vi "jfcRigControlOnly_v8.vi"() -> ()   [LabVIEW 2018]
doc: "The Low-Level Grab VI configures the number of buffers to use for the acquisition and configures an event callback to handle every other acquired image. A grab is appropriate for high-speed applications in which you need to process only one image at a time."
uses:
  jfcStateEnumWithBeep.ctl
  jfcOptoStateEnum.ctl
  65be267c-4a08-44b7-a786-4a83c3a2bfd1.vi
  <vilib>/DAQmx/write.llb/DAQmx Write (Digital Bool 1Line 1Point).vi
  <vilib>/DAQmx/write.llb/DAQmx Write (Analog 1D DBL 1Chan NSamp).vi
  <vilib>/DAQmx/read.llb/DAQmx Read (Analog 1D Wfm NChan NSamp).vi
  <vilib>/DAQmx/write.llb/DAQmx Write (Analog Wfm 1Chan NSamp).vi
  <vilib>/DAQmx/configure/timing.llb/DAQmx Timing (Sample Clock).vi
  <vilib>/Instr/_visa.llb/VISA Configure Serial Port (Instr).vi
  <vilib>/DAQmx/create/channels.llb/DAQmx Create Channel (DO-Digital Output).vi
  <vilib>/DAQmx/miscellaneous.llb/DAQmx Fill In Error Info.vi
  <vilib>/DAQmx/create/channels.llb/DAQmx Create Channel (CO-Pulse Generation-Frequency).vi
  <vilib>/DAQmx/configure/timing.llb/DAQmx Timing (Implicit).vi
  <vilib>/Waveform/WDTOps.llb/WDT Append Waveforms DBL.vi
  <resource>/objmgr/daqmx.rc
  <vilib>/measure/NI_MABase.lvlib
panel:
  out "State":T1
  in  "amplitude":dbl=2.0 step=0.5 format="%#_13g"
  in  "rampUpOpto":bool
  in  "optoMaxTime":dbl=60.0 format="%.1g"
  in  "opto every trial?":bool
  in  "InhOptoOffset":dbl=2.3 step=0.5 format="%#_13g"
  out "platformExtended":bool
  out "opto time":dbl
  out "trial / jump #":i32
  out "opto trial list":bool[](array[boolean])
  in  "seconds to wait at end":i32=30
  in  "manual opto ON\n(overides enable)":bool
  in  "Opto-inhibition \nwaveform?":bool=TRUE
  out "BeepOn":bool
  out "beepTimeCurrent":u32 caption="Elapsed Time (s)"
  out "beepTimeElapsed":bool caption="Time has Elapsed"
  out "Waveform Graph":waveform(dbl)(graph) caption="Optostim waveform"
  out "optostim on":bool
  out "cold air status":bool
  out "session time elapsed":bool
  in  "seconds to wait at beg":i32=30
  in  "constant seconds to wait":u32=10
  out "seconds elapsed":i32
  out "Waveform Chart":waveform(dbl)[](graph)=[{"t0"=timestamp(3694175544.180511 s since 1904-01-01), "dt"=9.999999999999999e-05, "Y"=[2.549736107551297, 2.547978168445268, 2.549816013874609, 2.5507748897564566, 2.5496562012280126, 2.548697325350701, 2.5489370443196644, 2.5513342340226637, 2.550934702403809, 2.54845760638198, 2.548697325350701, 2.5504552644620753, 2.5508547960801193, 2.549736107551297, 2.54845760638198, 2.549176763288871, 2.551893578290195, 2.550615077109212, 2.547978168445268, 2.5492566696119936], "attributes"=variant("NI_ChannelName"=variant(string "jumpVoltageInput6281"), "NI_UnitDescription"=variant(string "Volts"))}]
  out "# frames triggered":i32
  in  "seconds to record":i32=1200
  in  "Frames Per Second":dbl=400.0 format="%.1f"
  out "numSamplesAvg":i32=20
  in  "jumpThresh":dbl=2.8000000000000003 step=0.01 format="%_3g"
  in  "manual solenoid override":bool
  out "beenStopped":bool=TRUE
  in  "ExtensionLength (mm)":dbl=100.0 caption="Extension Length (mm)"
  out "jump voltage":dbl=2.549672182495309 format="%#_3g"
  in  "optostim enable":bool=TRUE
  out "error out":errorcluster={"status"=FALSE, "code"=1073676294, "source"="VISA Read in usbSimpleRelayCommand.vi->jfcRigControlOnly_v3_constantTimingWithBeep.vi"}
  in  "stop":bool
  # "optostim Enable"
  # "[change # frames \nin video program too]"
  # "----------------------------------------------------------------------------------------------------------------------------"
  # "5"
  # "10"
  # "15"
  # "20"
  # "25"
  # "30"
  # "35"
  # "40"
  # "45"
  # "50"
  # "55"
  # "60"
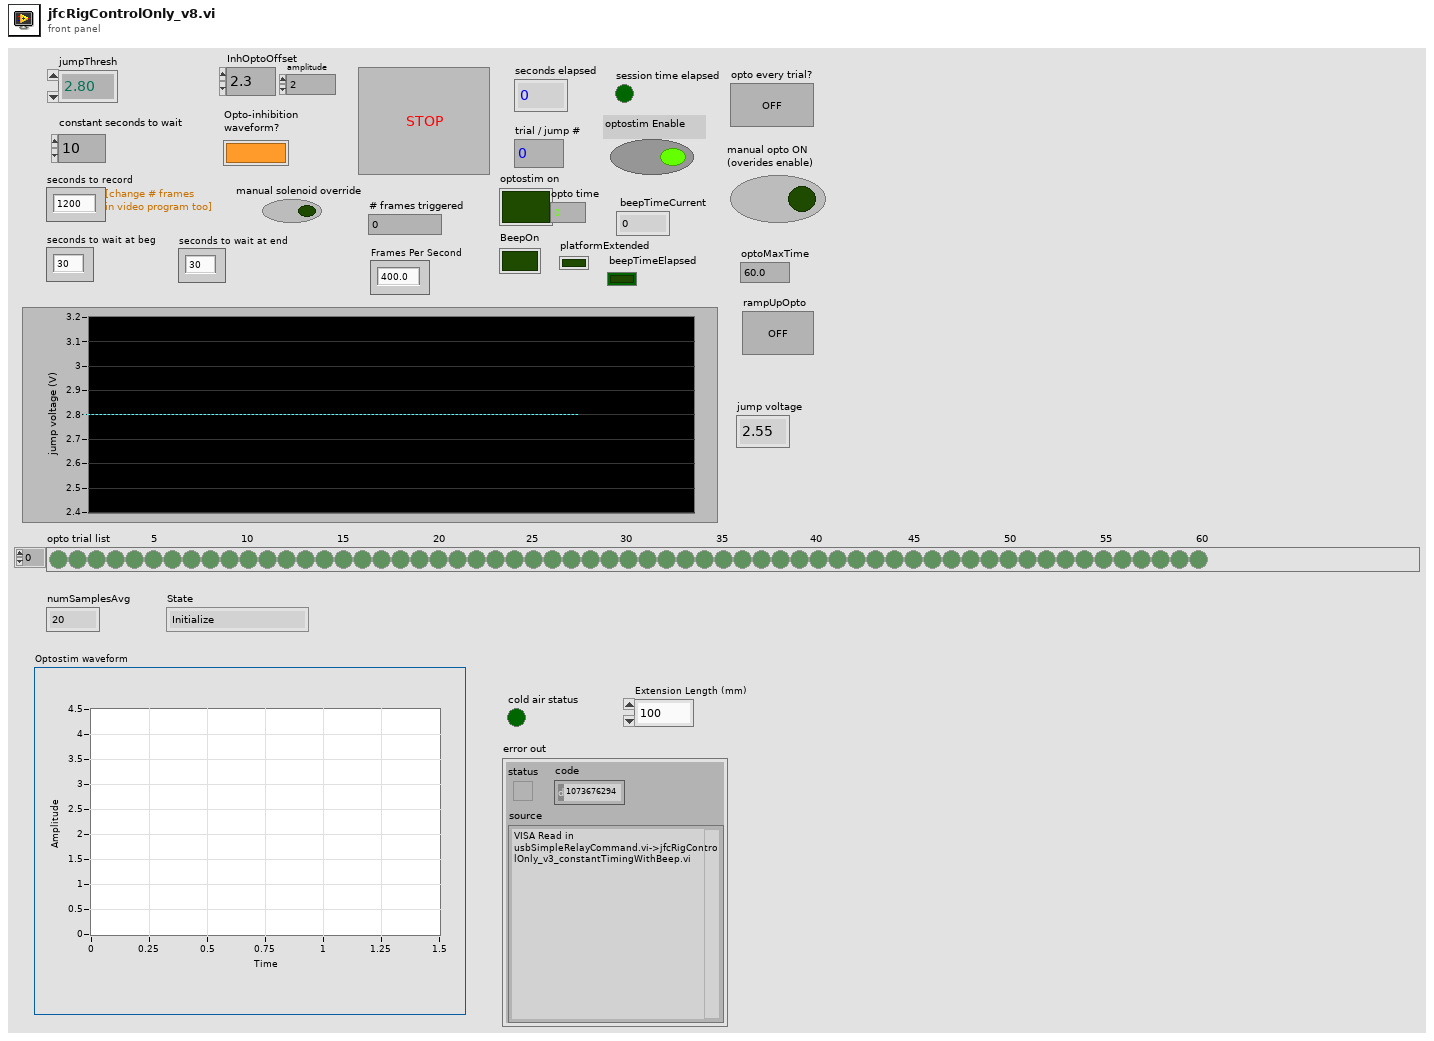
[diagram p1: front panel]
types:
  T1 = typedef "jfcStateEnumWithBeep.ctl" = enum16{"Initialize", "Reinitialize after jump", "Beep", "Wait for Thresh or Stop", "Turn Off Air and Reset Lever", "Wait after time elapsed", "Stop"}
  T2 = enum16{"Sine Wave", "Triangle Wave", "Square Wave", "Sawtooth Wave"}
  T3 = typedef "jfcOptoStateEnum.ctl" = enum16{"writeZeroVoltage", "WaitForStartOpto", "RampUpOpto", "OptoOn", "RampDownOpto"}
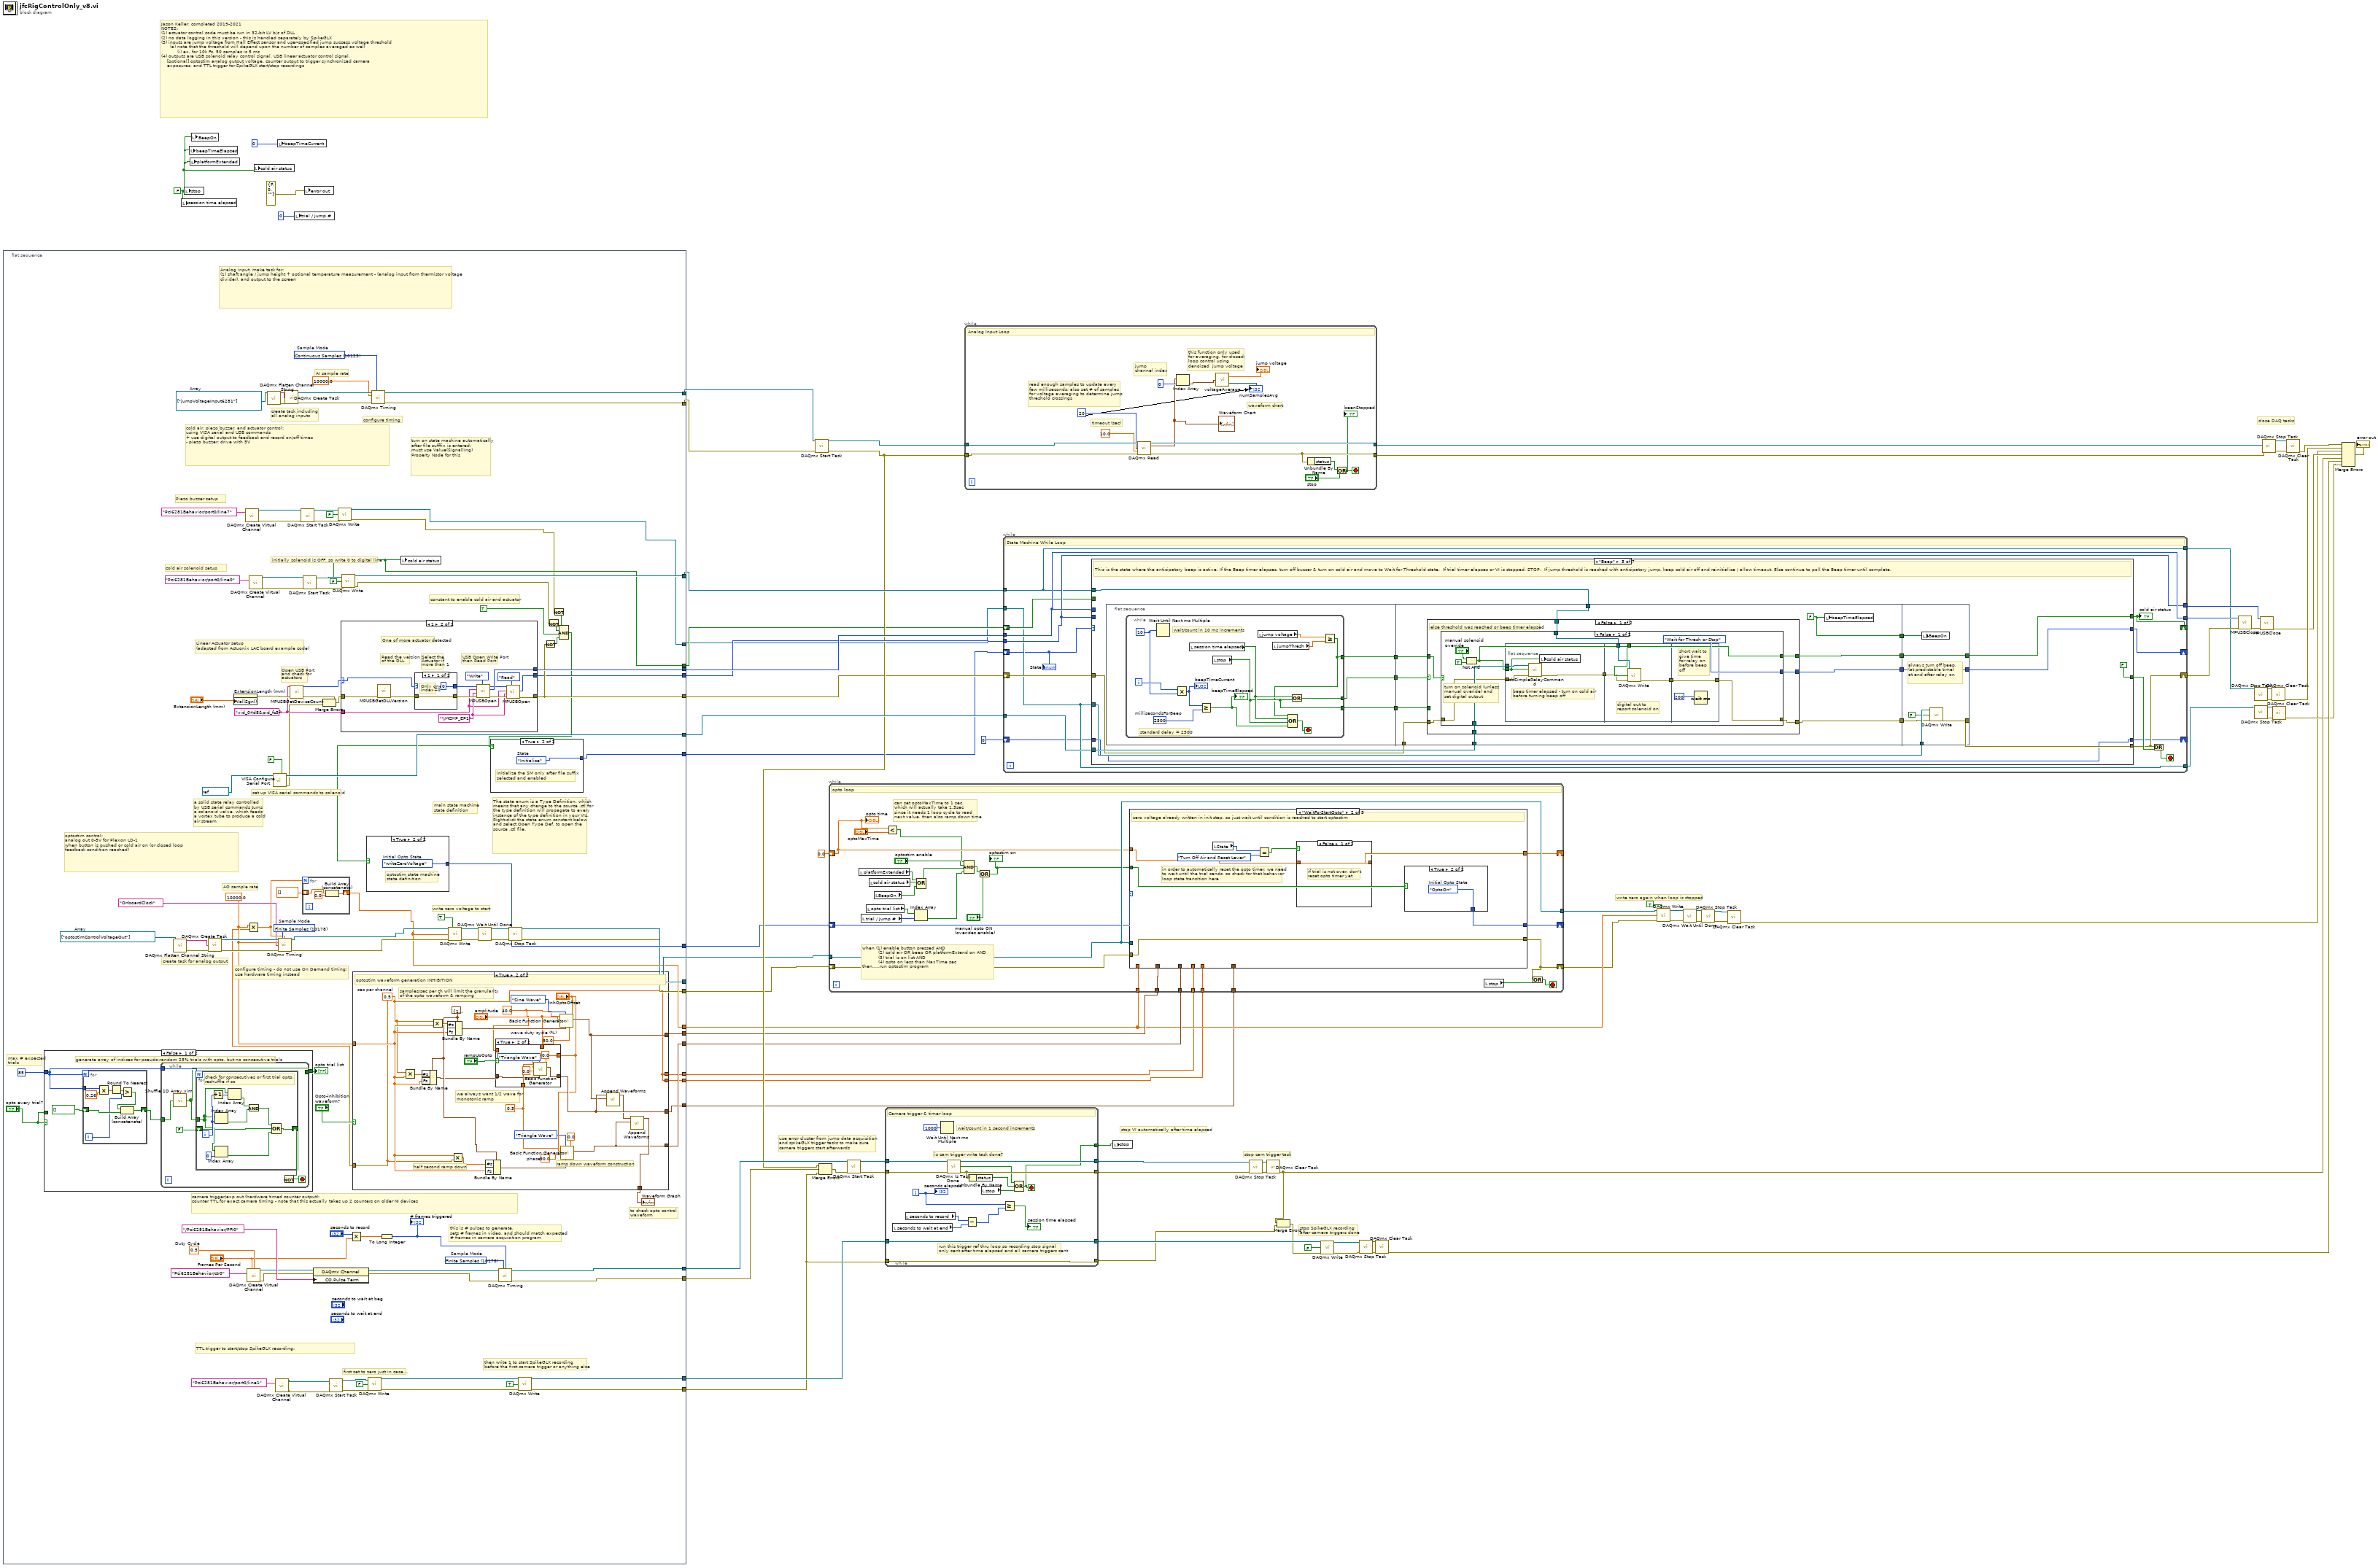
[diagram p0: block diagram]
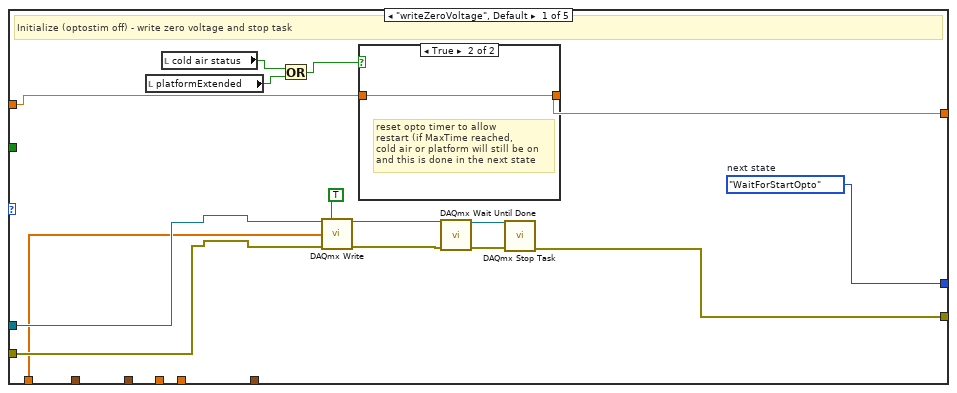
[diagram p2: hidden frame]
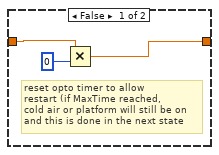
[diagram p3: hidden frame]
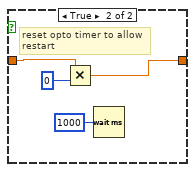
[diagram p4: hidden frame]
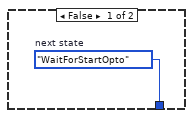
[diagram p5: hidden frame]
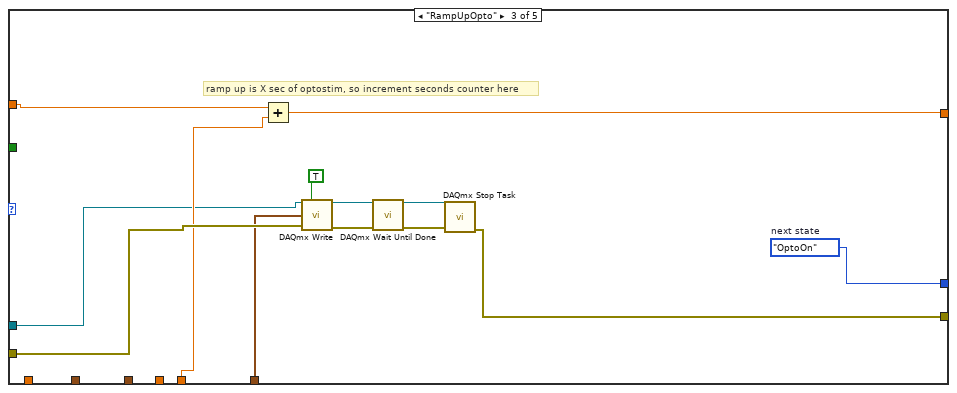
[diagram p6: hidden frame]
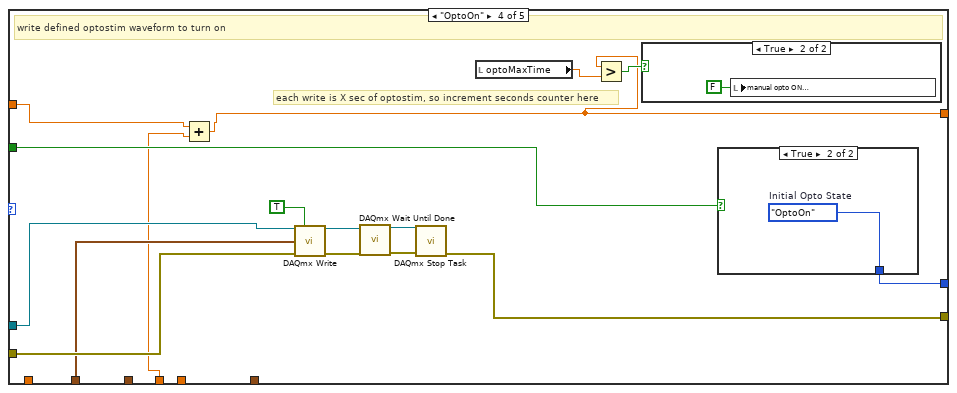
[diagram p7: hidden frame]
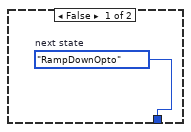
[diagram p9: hidden frame]
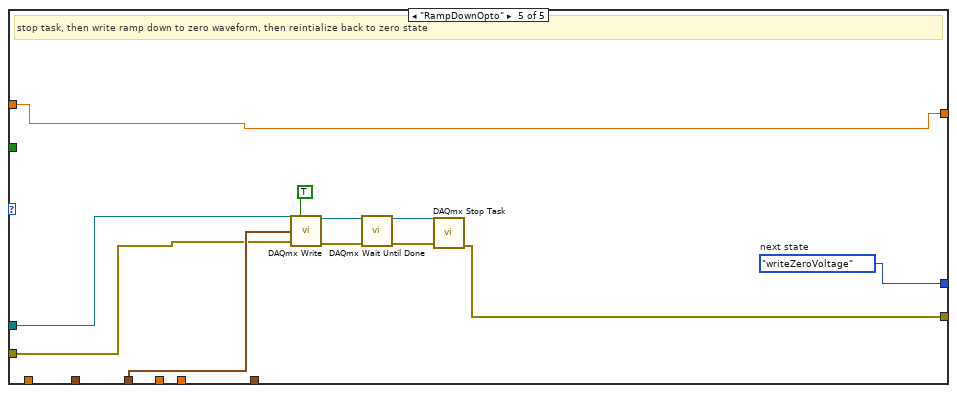
[diagram p10: hidden frame]
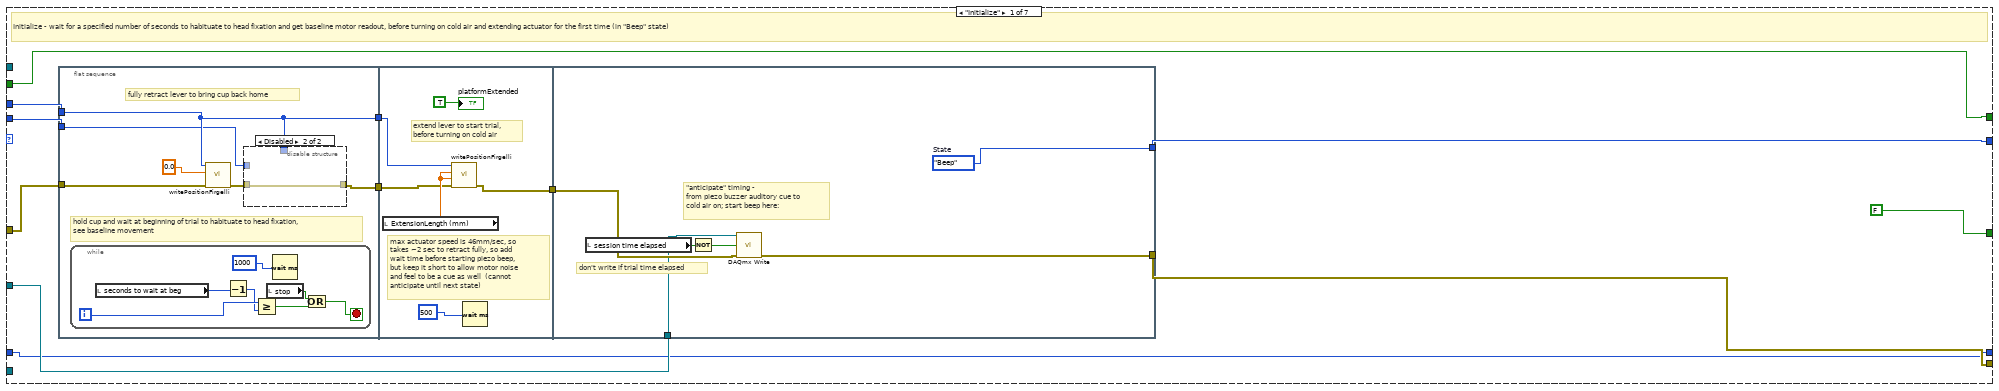
[diagram p11: hidden frame]
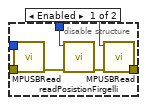
[diagram p12: hidden frame]
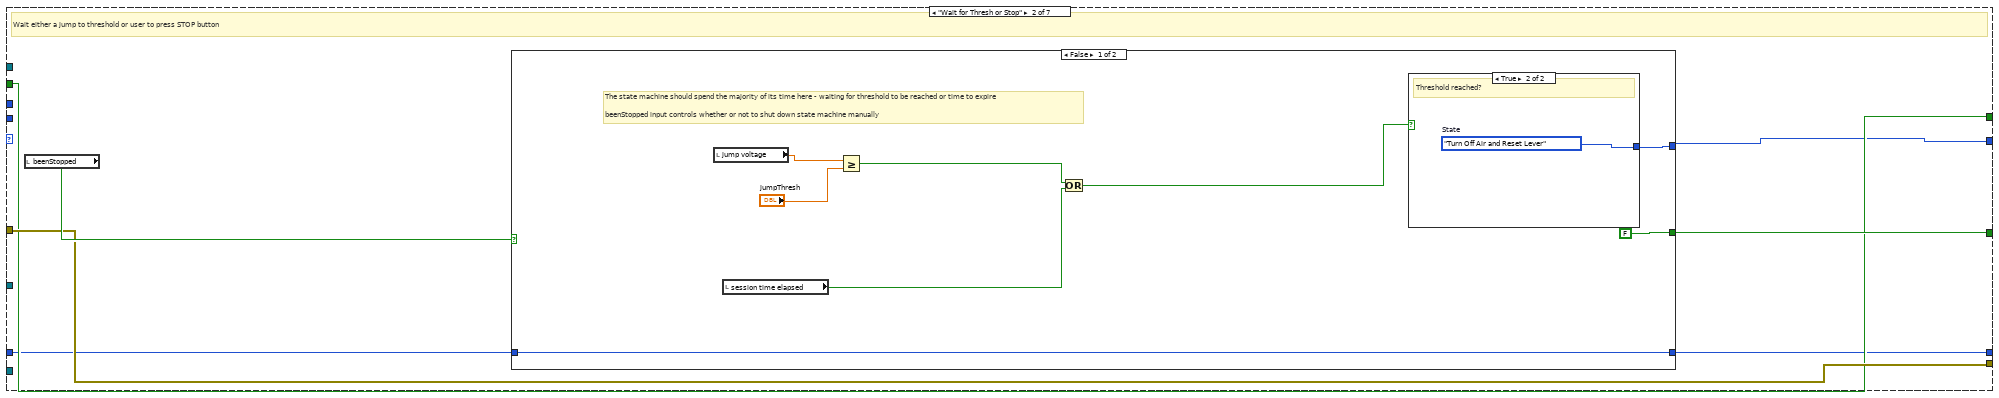
[diagram p13: hidden frame]
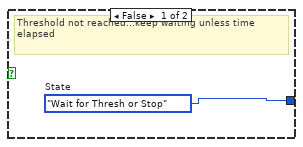
[diagram p14: hidden frame]
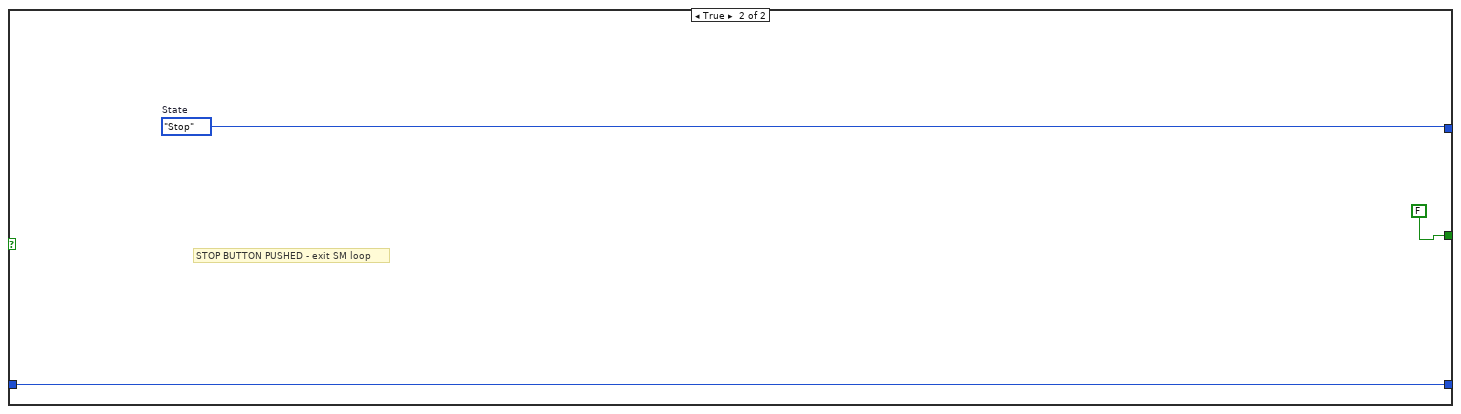
[diagram p15: hidden frame]
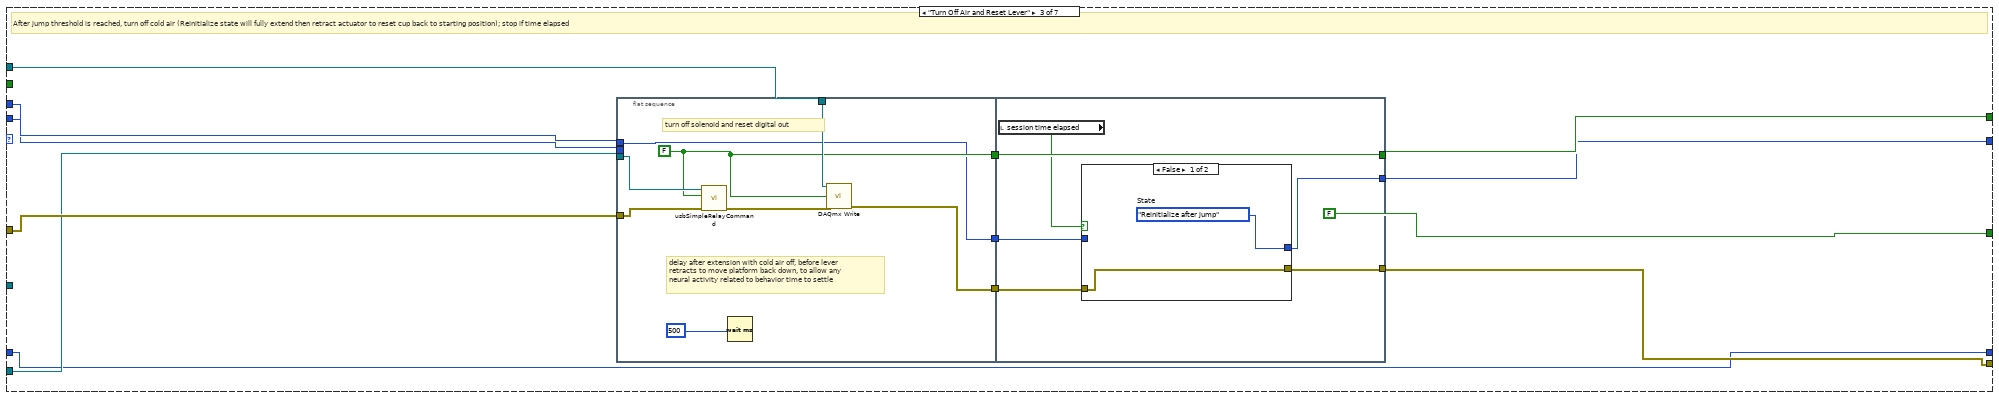
[diagram p16: hidden frame]
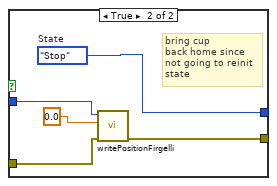
[diagram p17: hidden frame]
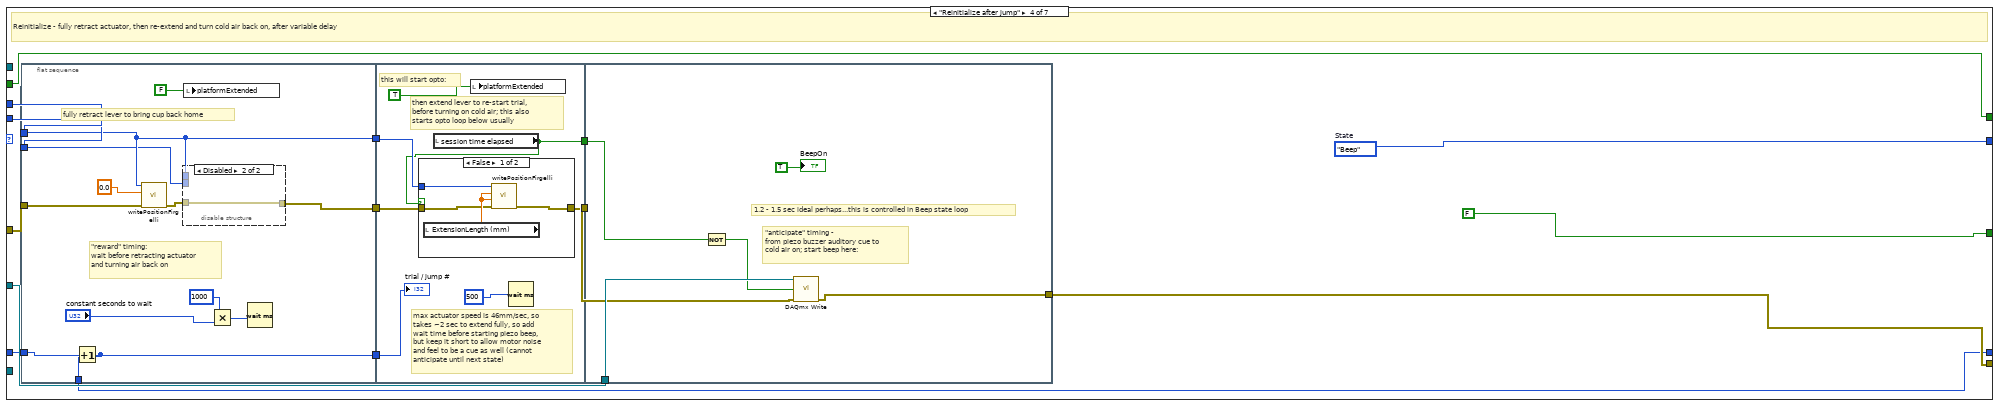
[diagram p18: hidden frame]
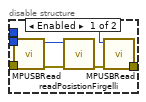
[diagram p19: hidden frame]
diagram:
  w4 = FALSE ("stop")
  # "stop cam trigger task"
  # "write zero again when loop is stopped"
  # "stop SpikeGLX recording\nafter camera triggers done"
  # "stop VI automatically after time elapsed"
  # "use error cluster from jump data acquisition\nand spikeGLX trigger tasks to make sure \ncamera triggers start afterwards"
  # "Jason Keller, completed 2019-2021\nNOTES: \n(1) actuator control code must be run in 32-bit LV b/c of DLL \n(2) no data logging in this version - this is handled separately by SpikeGLX\n(3) inputs are jump voltage from Hall Effect sensor and user-specified jump success voltage threshold\n      (a) note that the threshold will depend upon the number of samples averaged as well\n           (i) ex. for 10k Fs, 50 samples is 5 ms\n(4) outputs are USB solenoid relay control signal, USB linear actuator control signal, \n    [optional] optostim analog output voltage, counter output to trigger synchronized camera \n    exposures, and TTL trigger for SpikeGLX start/stop recordings"
  # "close DAQ tasks"
  n1 = flat-sequence {
    tunnel: [w150] -> w71
    tunnel: [w149] -> w70
    tunnel: [w162] -> w60
    tunnel: [w173] -> w19
    tunnel: [w168] -> w69
    tunnel: [w167] -> w48
    tunnel: [w165] -> w67
    tunnel: [w158] -> w59
    tunnel: [w136] -> w52
    tunnel: [w135] -> w50
    tunnel: [w134] -> w47
    tunnel: [w115] -> w44
    tunnel: [w92] -> w43
    tunnel: [w127] -> w46
    tunnel: [w126] -> w45
    tunnel: [w125] -> w40
    tunnel: [w117] -> w38
    tunnel: [w104] -> w36
    tunnel: [w103] -> w35
    tunnel: [w97] -> w24
    tunnel: [w89] -> w2
    tunnel: [w88] -> w3
    tunnel: [w87] -> w1
    frame #0 {
      w148 = 0.5  # Duty Cycle
      w128 = refnum<k21>[] ["optostimControlVoltageOut"]  # Array
      w86 = 10000.0 ("Sample Rate")
      w132 = 10178 items=["Finite Samples"=10178, "Continuous Samples"=10123, "Hardware Timed Single Point"=12522]  # Sample Mode
      w141 = 10178 items=["Finite Samples"=10178, "Continuous Samples"=10123, "Hardware Timed Single Point"=12522]  # Sample Mode
      w134 = FALSE ("data")
      w169 = "vid_04d8&pid_fc5f"
      w174 = refnum<k21>[] ["jumpVoltageInput6281"]  # Array
      w179 = 10123 items=["Finite Samples"=10178, "Continuous Samples"=10123, "Hardware Timed Single Point"=12522]  # Sample Mode
      # "max # expected\ntrials"
      # "to check opto control\nwaveform"
      # "cold air solenoid setup"
      # "Piezo buzzer setup"
      # "Piezo buzzer setup"
      # "then write 1 to start SpikeGLX recording\nbefore the first camera trigger or anything else"
      # "first set to zero just in case..."
      # "TTL trigger to start/stop SpikeGLX recording:"
      # "write zero voltage to start"
      # "AO sample rate"
      # "create task for analog output"
      # "configure timing - do not use On Demand timing; \nuse hardware timing instead"
      # "this is # pulses to generate,\nsets # frames in video, and should match expected \n# frames in camera acquisition program"
      # "camera trigger/exp out (hardware timed counter output): \ncounter TTL for exact camera timing - note that this actually takes up 2 counters on older NI devices"
      # "initially solenoid is OFF, so write 0 to digital line"
      # "set up VISA serial commands to solenoid"
      # "Linear Actuator setup\n(adapted from Actuonix LAC board example code)"
      # "Open USB Port\nand check for\nactuators"
      # "turn on state machine automatically\nafter file sufffix is entered;\nmust use Value(Signalling) \nProperty Node for this"
      # "The state enum is a Type Definition, which means that any change to the source .ctl for the type definition will propagate to every instance of the type definition in your VIs. Right-click the state enum constant below and select Open Type Def. to open the source .ctl file."
      # "main state machine\nstate definition"
      # "a solid state relay controlled\nby USB serial commands turns\na solenoid valve, which feeds\na vortex tube to produce a cold\nair stream"
      # "AI sample rate"
      # "create task including\nall analog inputs"
      # "configure timing"
      # "constant to enable cold air and actuator"
      # "optostim control: \nanalog out 0-5V for Plexon LD-1\nwhen button is pushed or cold air on (or closed loop \nfeedback condition reached)"
      # "Analog input, make task for:\n(1) shaft angle / jump height + optional temperature measurement - (analog input from thermistor voltage divider), and output to the screen"
      # "cold air, piezo buzzer, and actuator control: \nusing VISA serial and USB commands\n+ use digital output to feedback and record on/off times\n- piezo buzzer: drive with 5V"
      n2 = case shown="False" "opto every trial?" {
        tunnel: 85 -> [w182 w212]
        tunnel: [w181 w208] -> w90
        tunnel: "opto every trial?" -> [_ w213]
        frame False {
          # "generate array of indices for pseudo-random 25% trials with opto, but no consecutive trials"
          n3 = for {
            N: w182 -> [_]
            shift-right: [w188] -> w183
            shift-left: bool[] [] -> [w189]
            tunnel: w182 -> [w191]
            i -> [w184]
            n4 = Multiply(x=w191, y=0.26) -> (x*y=w186:dbl)
            n5 = Round To Nearest(number=w186) -> (nearest integer value=w185:dbl)
            n6 = Greater?(x=w185, y=w184) -> (0:w190:bool)
            n7 = Build Array (concatenate)(w190, w189) -> (w188:bool[])
          }
          n8 = while {
            tunnel: w183 -> [w197]
            tunnel: w182 -> [w196]
            tunnel: [w192] -> w181
            stop <- w194 stop-if-true
            n9 = call "Shuffle 1D Array.vim"("array"=w197) -> ("shuffled array"=w192:bool[])  [unwired: 4 in]
            n10 = for {
              N: w196 -> [_]
              tunnel: w192 -> [w202]
              shift-right: [w200] -> w193
              shift-left: FALSE -> [w201]
              i -> [w206]
              # "check for consecutives or first trial opto, \nreshuffle if so"
              n11 = Increment(x=w206) -> (x+1=w207:i32)
              n12 = Index Array(array=w202, index=w206) -> (element=w204:bool)
              n13 = Index Array(array=w202, index=0) -> (element=w198:bool)
              n14 = Index Array(array=w202, index=w207) -> (element=w205:bool)
              n15 = And(x=w205, y=w204) -> (x .and. y?=w199:bool)
              n16 = Compound Arithmetic op=OR(w199, w201, w198) -> (w200:bool)
            }
            n17 = Not(x=w193) -> (.not. x?=w194:bool)
          }
        }
        frame True {
          # "all trials except for #0"
          n18 = Decrement(x=w212) -> (x-1=w211:i32)
          n19 = Initialize Array(w213, w211) -> (w209:bool[])
          n20 = Build Array (concatenate)(FALSE, w209) -> (w208:bool[])
        }
      }
      "opto trial list" <- w90
      n21 = call <vilib>:"DAQmx Flatten Channel String.vi"("names in"=w128) -> ("names out"=w129:string, "error out"=w130:errorcluster)  [unwired: 13 in]
      n22 = call <vilib>:"DAQmx Create Task.vi"("global virtual channels"=w129, "error in"=w130) -> ("task out"=w131:refnum<k21>, "error out"=w93:errorcluster)  [unwired: 12 in]
      n23 = property on="ExtensionLength (mm)" class="DigNum (strict)"("Val(Sgnl)"="ExtensionLength (mm)") -> (error out=w172:errorcluster)  [unwired: 2 in, 1 out]
      n24 = call-poly <vilib>:"DAQmx Create Virtual Channel.vi"("lines"=tag "Pci6281Behavior/port0/line7") -> ("task out"=w82:refnum<k21>, "error out"=w81:errorcluster)  [unwired: 13 in]
      n25 = call-poly <vilib>:"DAQmx Create Virtual Channel.vi"("frequency"="Frames Per Second", "duty cycle"=w148, "counter"=tag "Pci6281Behavior/ctr0" ("Counter")) -> ("task out"=w143:refnum<k21>, "error out"=w144:errorcluster)  [unwired: 11 in]
      n26 = call-poly <vilib>:"DAQmx Create Virtual Channel.vi"("lines"=tag "Pci6281Behavior/port0/line0") -> ("task out"=w80:refnum<k21>, "error out"=w79:errorcluster)  [unwired: 13 in]
      n27 = call <vilib>:"DAQmx Flatten Channel String.vi"("names in"=w174) -> ("names out"=w175:string, "error out"=w176:errorcluster)  [unwired: 13 in]
      n28 = call-poly "VISA Configure Serial Port"("VISA resource name"=refnum<visa-resource-name> "COM4" ("relay COM port"), "Enable Termination\nChar (T)"=FALSE ("Enable Termination\nChar (T)")) -> ("VISA resource name out"=w162:refnum<visa-resource-name>, "error out"=w161:errorcluster)  [unwired: 12 in]
      n29 = call-poly <vilib>:"DAQmx Create Virtual Channel.vi"("lines"=tag "Pci6281Behavior/port0/line1") -> ("task out"=w111:refnum<k21>, "error out"=w110:errorcluster)  [unwired: 13 in]
      n30 = call <vilib>:"DAQmx Create Task.vi"("global virtual channels"=w175, "error in"=w176) -> ("task out"=w178:refnum<k21>, "error out"=w177:errorcluster)  [unwired: 12 in]
      n31 = call "MPUSBGetDeviceCount.vi"("error in (no error)"=w172, "pVID_PID"=w169) -> ("error out"=w160:errorcluster, "return_value"=w171:u32)  [unwired: 8 out]
      n32 = call <vilib>:"DAQmx Start Task.vi"("task/channels in"=w82, "error in"=w81) -> ("task out"=w98:refnum<k21>, "error out"=w101:errorcluster)  [unwired: 12 in]
      n33 = call <vilib>:"DAQmx Start Task.vi"("task/channels in"=w80, "error in"=w79) -> ("task out"=w154:refnum<k21>, "error out"=w153:errorcluster)  [unwired: 12 in]
      n34 = property class="DAQmx Channel"(reference=w143, error in=w144, "CO.Pulse.Term"=tag "/Pci6281Behavior/PFI0" ("Output Terminal")) -> (reference out=w147:refnum<k21>, error out=w146:errorcluster)
      n35 = Merge Errors(w160, w161) -> (w159:errorcluster)
      n36 = call <vilib>:"DAQmx Start Task.vi"("task/channels in"=w111, "error in"=w110) -> ("task out"=w113:refnum<k21>, "error out"=w112:errorcluster)  [unwired: 12 in]
      n37 = call-poly <vilib>:"DAQmx Write.vi"("task/channels in"=w98, "data"=FALSE, "error in"=w101) -> ("task out"=w97:refnum<k21>, "error out"=w96:errorcluster)  [unwired: 10 in, 1 out]
      n38 = case shown="1" w171 {
        selector: w171 -> [_ w282]
        tunnel: w159 -> [w272 w284]
        tunnel: w169 -> [_ w278]
        tunnel: [u32 0 ("HANDLE") w283] -> w168
        tunnel: [w272 w277] -> w167
        tunnel: [u32 0 ("HANDLE") w276] -> w165
        frame 0, Default {
          # "No actuator detected"
        }
        frame 1 {
          w279 = "\\MCHP_EP1" ("pEP")
          # "One of more actuator detected"
          # "Select the\nActuator if\nmore than 1"
          # "Read the version\nof the DLL"
          # "USB Open Write Port\nthen Read Port"
          n39 = call "MPUSBGetDLLVersion.vi"("error in (no error)"=w284) -> ("error out"=w287:errorcluster)  [unwired: 10 out]
          n40 = case shown="1" w282 {
            selector: w282 -> [_ w291]
            tunnel: w287 -> [w290 w294]
            tunnel: [w290 w293] -> w286
            tunnel: [u32 0 ("Selected") w292] -> w285
            frame 1 {
              # "Only one\nIndex=0"
            }
            frame Default {
              n41 = call "actuatorSelect.vi"("error in (no error)"=w294, "Devices"=w291) -> ("error out"=w293:errorcluster, "Selected"=w292:u32)  [unwired: 8 out]
            }
          }
          n42 = call "MPUSBOpen.vi"("dwDir"=enum16{"Write", "Read"}."Write", "error in (no error)"=w286, "pEP"=w279, "pVID_PID"=w278, "instance"=w285) -> ("error out"=w280:errorcluster, "HANDLE"=w283:u32, "instanceOut"=w275:u32)  [unwired: 4 in]
          n43 = call "MPUSBOpen.vi"("dwDir"=enum16{"Write", "Read"}."Read", "error in (no error)"=w280, "pEP"=w279, "pVID_PID"=w278, "instance"=w275) -> ("error out"=w277:errorcluster, "HANDLE"=w276:u32)  [unwired: 3 in, 2 out]
        }
      }
      n44 = call-poly <vilib>:"DAQmx Write.vi"("task/channels in"=w154, "data"=w134, "error in"=w153) -> ("task out"=w158:refnum<k21>, "error out"=w157:errorcluster)  [unwired: 10 in, 1 out]
      n45 = Multiply(x="seconds to record", y="Frames Per Second") -> (x*y=w138:dbl)
      n46 = case shown="True" "Opto-inhibition \nwaveform?" {
        tunnel: w86 -> [w222 w240]
        tunnel: [w227 w243] -> w126
        tunnel: [w224 w241] -> w125
        tunnel: [w225 w247] -> w94
        tunnel: [w217 w232] -> w89
        tunnel: [w217 w232] -> w88
        tunnel: [w228 w244] -> w87
        tunnel: [w217 w232] -> w84
        frame False {
          w217 = 0.5  # sec per channel
          w223 = 40.0 ("y")
          w218 = T2."Square Wave" ("signal type")
          w219 = 2.5  # amplitude
          w229 = 2.5  # offset
          w221 = 20.0  # square wave duty cycle (%)
          w220 = cluster{"Fs":dbl, "#s":dbl} {"Fs"=1000.0, "#s"=1000.0} ("sampling info")
          # "samples /sec per ch will limit the granularity\nof the opto waveform & ramping"
          # "excitation waveform\nex. 40Hz, 5ms pulse width"
          # "ex. 10ms/25ms = 0.4"
          # "optostim waveform generation EXCITATION"
          n47 = Multiply(x=w217, y=w222) -> (x*y=w231:dbl)
          n48 = Bundle By Name(cluster=w220, "#s"=w231, "Fs"=w222) -> (w230:cluster{"Fs":dbl, "#s":dbl})
          n49 = call <vilib>:"Basic Function Generator.vi"("offset"=w229, "square wave duty cycle (%)"=w221, "sampling info"=w230, "signal type"=w218, "amplitude"=w219, "frequency"=w223) -> ("signal out"=w227:waveform(dbl))  [unwired: 3 in, 2 out]
          n50 = call "buildRampDownWaveform.vi"("Fs"=w222, "square wave duty cycle (%)"=w221, "signal type"=w218, "input cluster"=w220, "amplitude"=w219, "freq"=w223, "sec rampdown"=w217) -> ("rampDown out"=w224:waveform(dbl))  [unwired: 4 in]
          n51 = call "buildRampUpWaveform.vi"("Fs"=w222, "square wave duty cycle (%)"=w221, "signal type"=w218, "input cluster"=w220, "amplitude"=w219, "freq"=w223, "sec rampup"=w217) -> ("rampUp out"=w228:waveform(dbl))  [unwired: 4 in]
          n52 = call-poly <vilib>:"Append Waveforms.vi"("waveform B"=w227, "waveform A"=w228) -> ("waveform out"=w226:waveform(dbl))  [unwired: 8 in, 1 out]
          n53 = call-poly <vilib>:"Append Waveforms.vi"("waveform B"=w224, "waveform A"=w226) -> ("waveform out"=w225:waveform(dbl))  [unwired: 8 in, 1 out]
        }
        frame True {
          w232 = 0.5  # sec per channel
          w234 = 0.5 ("frequency")
          w233 = 40.0 ("frequency")
          w254 = 90.0  # phase
          w255 = 50.0  # wave duty cycle (%)
          w246 = cluster{"Fs":dbl, "#s":dbl} {"Fs"=1000.0, "#s"=1000.0} ("sampling info")
          # "half second ramp down"
          # "samples/sec per ch will limit the granularity\nof the opto waveform & ramping"
          # "we always want 1/2 wave for\nmonotonic ramp"
          # "ramp down waveform construction"
          # "optostim waveform generation INHIBITION"
          n54 = Multiply(x=w232, y=w240) -> (x*y=w239:dbl)
          n55 = Bundle By Name(cluster=w246, "#s"=w239, "Fs"=w240) -> (w245:cluster{"Fs":dbl, "#s":dbl})
          n56 = Multiply(x=w232, y=w240) -> (x*y=w250:dbl)
          n57 = Bundle By Name(cluster=w246, "#s"=w250, "Fs"=w240) -> (w249:cluster{"Fs":dbl, "#s":dbl})
          n58 = Multiply(x=w240, y=w232) -> (x*y=w251:dbl)
          n59 = Bundle By Name(cluster=w246, "#s"=w251, "Fs"=w240) -> (w253:cluster{"Fs":dbl, "#s":dbl})
          n60 = case shown="True" "rampUpOpto" {
            tunnel: w245 -> [w262 w264]
            tunnel: [w260 w263] -> w244
            tunnel: "InhOptoOffset" -> [w258 w267]
            tunnel: "amplitude" -> [w257 _]
            tunnel: w233 -> [w256 _]
            tunnel: w234 -> [_ w269]
            frame False {
              w261 = 0.0  # phase
              n61 = call <vilib>:"Basic Function Generator.vi"("offset"=w258, "sampling info"=w262, "signal type"=T2."Sine Wave", "phase"=w261, "amplitude"=w257, "frequency"=w256) -> ("signal out"=w260:waveform(dbl))  [unwired: 3 in, 2 out]
            }
            frame True {
              n62 = call <vilib>:"Basic Function Generator.vi"("offset"=0.0, "sampling info"=w264, "signal type"=T2."Triangle Wave", "phase"=0.0, "amplitude"=w267, "frequency"=w269) -> ("signal out"=w263:waveform(dbl))  [unwired: 3 in, 2 out]
            }
          }
          n63 = call <vilib>:"Basic Function Generator.vi"("offset"="InhOptoOffset", "square wave duty cycle (%)"=w255, "sampling info"=w249, "signal type"=T2."Sine Wave", "amplitude"="amplitude", "frequency"=w233) -> ("signal out"=w243:waveform(dbl))  [unwired: 3 in, 2 out]
          n64 = call <vilib>:"Basic Function Generator.vi"("offset"=0.0, "sampling info"=w253, "signal type"=T2."Triangle Wave", "phase"=w254, "amplitude"="InhOptoOffset", "frequency"=w234) -> ("signal out"=w241:waveform(dbl))  [unwired: 3 in, 2 out]
          n65 = call-poly <vilib>:"Append Waveforms.vi"("waveform B"=w243, "waveform A"=w244) -> ("waveform out"=w242:waveform(dbl))  [unwired: 8 in, 1 out]
          n66 = call-poly <vilib>:"Append Waveforms.vi"("waveform B"=w241, "waveform A"=w242) -> ("waveform out"=w247:waveform(dbl))  [unwired: 8 in, 1 out]
        }
      }
      "Waveform Graph" <- w94
      n67 = Multiply(x=w86, y=w84) -> (x*y=w85:dbl)
      n68 = call-poly <vilib>:"DAQmx Timing.vi"("task/channels in"=w131, "sample mode"=w132, "samples per channel"=w85, "rate"=w86, "source"=tag "OnboardClock", "error in"=w93) -> ("task out"=w122:refnum<k21>, "error out"=w123:errorcluster)  [unwired: 8 in]
      n69 = for {
        N: w85 -> [_]
        shift-right: [w216] -> w117
        shift-left: dbl[] [] -> [w214]
        n70 = Build Array (concatenate)(w214, 0.0 ("element")) -> (w216:dbl[])
      }
      n71 = call-poly <vilib>:"DAQmx Write.vi"("task/channels in"=w113, "data"=FALSE, "error in"=w112) -> ("task out"=w106:refnum<k21>, "error out"=w105:errorcluster)  [unwired: 10 in, 1 out]
      n72 = call-poly <vilib>:"DAQmx Timing.vi"("task/channels in"=w178, "sample mode"=w179, "rate"=10000.0 ("Sample Rate"), "error in"=w177) -> ("task out"=w150:refnum<k21>, "error out"=w149:errorcluster)  [unwired: 10 in]
      n73 = To Long Integer(number=w138) -> (32bit integer=w137:i32)
      "# frames triggered" <- w137
      n74 = local write "cold air status"(w134) -> ()
      n75 = call-poly <vilib>:"DAQmx Write.vi"("task/channels in"=w122, "auto start"=TRUE, "data"=w117, "error in"=w123) -> ("task out"=w120:refnum<k21>, "error out"=w119:errorcluster)  [unwired: 9 in, 1 out]
      n76 = call <vilib>:"DAQmx Wait Until Done.vi"("task/channels in"=w120, "error in"=w119) -> ("task out"=w116:refnum<k21>, "error out"=w114:errorcluster)  [unwired: 12 in]
      n77 = call-poly <vilib>:"DAQmx Timing.vi"("task/channels in"=w147, "sample mode"=w141, "samples per channel"=w137, "error in"=w146) -> ("task out"=w135:refnum<k21>, "error out"=w136:errorcluster)  [unwired: 10 in]
      n78 = call <vilib>:"DAQmx Stop Task.vi"("task/channels in"=w116, "error in"=w114) -> ("task out"=w115:refnum<k21>, "error out"=w92:errorcluster)  [unwired: 12 in]
      n79 = call-poly <vilib>:"DAQmx Write.vi"("task/channels in"=w106, "data"=TRUE, "error in"=w105) -> ("task out"=w104:refnum<k21>, "error out"=w103:errorcluster)  [unwired: 10 in, 1 out]
      n80 = Not(x=w167) -> (.not. x?=w170:bool)
      n81 = Not(x=w157) -> (.not. x?=w156:bool)
      n82 = Not(x=w96) -> (.not. x?=w102:bool)
      n83 = Compound Arithmetic op=AND(w102, w156, TRUE ("Peltier Control"), w170) -> (w133:bool)
      n84 = case shown="True" w133 {
        tunnel: [w270 w271] -> w127
        frame False {
          w270 = jfcOptoStateEnum."writeZeroVoltage"  # Initial Opto State
        }
        frame True {
          w271 = jfcOptoStateEnum."writeZeroVoltage"  # Initial Opto State
          # "optostim state machine\nstate definition"
        }
      }
      n85 = case shown="True" w133 {
        tunnel: [w295 w296] -> w173
        frame False {
          w295 = jfcStateEnumWithBeep."Stop"  # State
          # "cold air and actuator disabled"
        }
        frame True {
          w296 = jfcStateEnumWithBeep."Initialize"  # State
          # "initialize the SM only after file suffix\nselected and enabled"
        }
      }
    }
  }
  n86 = local write "session time elapsed"(w4) -> ()
  n87 = local write "stop"(w4) -> ()
  n88 = local write "beepTimeElapsed"(w4) -> ()
  n89 = local write "platformExtended"(w4) -> ()
  n90 = local write "BeepOn"(w4) -> ()
  n91 = local write "cold air status"(w4) -> ()
  n92 = local write "beepTimeCurrent"(u32 0 ("beepTimeCurrent")) -> ()
  n93 = local write "trial / jump #"(0 ("trial / jump #")) -> ()
  n94 = local write "error out"(errorcluster {"status"=FALSE, "code"=0, "source"=""} ("error constant")) -> ()
  n95 = call <vilib>:"DAQmx Start Task.vi"("task/channels in"=w71, "error in"=w70) -> ("task out"=w78:refnum<k21>, "error out"=w49:errorcluster)  [unwired: 12 in]
  n96 = Merge Errors(w49, w52, w35) -> (w51:errorcluster)
  n97 = while "Opto while loop" {
    tunnel: w44 -> [w322]
    tunnel: [w322] -> w12
    tunnel: w45 -> [w321]
    shift-right: [w319] -> w8
    shift-left: w43 -> [w323]
    tunnel: w40 -> [w320]
    shift-right: [w315] -> _
    shift-left: w46 -> [w316]
    tunnel: w38 -> [w314]
    shift-right: [w304] -> _
    shift-left: 0.0 -> [w303]
    tunnel: w2 -> [w299]
    tunnel: w3 -> [w298]
    tunnel: w1 -> [w297]
    stop <- w317 stop-if-true
    # "can set optoMaxTime to 1 sec,\nwhich will actually take 1.5sec \nsince it needs 1 loop cycle to read\nnext value, then also ramp down time"
    # "when (1) enable button pressed AND \n           (2) cold air OR beep OR platformExtend on AND\n           (3) trial is on list AND\n           (4) opto on less than MaxTime sec\nthen.....run optostim program"
    # "opto loop"
    n98 = local read "platformExtended"() -> (w300:bool)
    n99 = local read "trial / jump #"() -> (w305:i32)
    n100 = local read "opto trial list"() -> (w307:bool[])
    n101 = local read "cold air status"() -> (w313:bool)
    n102 = local read "BeepOn"() -> (w312:bool)
    n103 = Less?(x=w303, y="optoMaxTime") -> (x < y?=w301:bool)
    n104 = Index Array(array=w307, index=w305) -> (element=w306:bool)
    n105 = Compound Arithmetic op=OR(w300, w313, w312) -> (w311:bool)
    n106 = Compound Arithmetic op=AND(w301, "optostim enable", w311, w306) -> (w310:bool)
    n107 = Or(x=w310, y="manual opto ON\n(overides enable)") -> (x .or. y?=w309:bool)
    "optostim on" <- w309
    n108 = case shown="\"WaitForStartOpto\"" w316 {
      tunnel: w322 -> [w336 _ w360 w387 w399]
      tunnel: w323 -> [w335 w350 w366 w386 w398]
      tunnel: w321 -> [_ _ _ w384 _]
      tunnel: [w331 w350 w361 w377 w392] -> w319
      tunnel: w320 -> [_ _ _ _ w401]
      tunnel: w309 -> [_ w351 _ w385 _]
      tunnel: [w337 w349 w362 w380 w397] -> w315
      tunnel: w314 -> [w334 _ _ _ _]
      tunnel: [w328 w347 w363 w373 w391] -> w304
      tunnel: w303 -> [w329 w348 w365 w376 w391]
      tunnel: w299 -> [_ _ w364 _ _]
      tunnel: w298 -> [_ _ _ w375 _]
      tunnel: w297 -> [_ _ w359 _ _]
      frame "writeZeroVoltage", Default {
        w337 = jfcOptoStateEnum."WaitForStartOpto"  # next state
        # "Initialize (optostim off) - write zero voltage and stop task"
        n109 = local read "platformExtended"() -> (w326:bool)
        n110 = local read "cold air status"() -> (w327:bool)
        n111 = Or(x=w327, y=w326) -> (x .or. y?=w325:bool)
        n112 = call-poly <vilib>:"DAQmx Write.vi"("task/channels in"=w336, "auto start"=TRUE, "data"=w334, "error in"=w335) -> ("task out"=w339:refnum<k21>, "error out"=w330:errorcluster)  [unwired: 9 in, 1 out]
        n113 = case shown="True" w325 {
          tunnel: w329 -> [w341 w343]
          tunnel: [w340 w343] -> w328
          frame False {
            # "reset opto timer to allow\nrestart (if MaxTime reached, \ncold air or platform will still be on \nand this is done in the next state"
            n114 = Multiply(x=w341, y=0) -> (x*y=w340:dbl)
          }
          frame True {
            # "reset opto timer to allow\nrestart (if MaxTime reached, \ncold air or platform will still be on \nand this is done in the next state"
          }
        }
        n115 = call <vilib>:"DAQmx Wait Until Done.vi"("task/channels in"=w339, "error in"=w330) -> ("task out"=w333:refnum<k21>, "error out"=w332:errorcluster)  [unwired: 12 in]
        n116 = call <vilib>:"DAQmx Stop Task.vi"("task/channels in"=w333, "error in"=w332) -> ("error out"=w331:errorcluster)  [unwired: 12 in, 1 out]
      }
      frame "WaitForStartOpto" {
        # "in order to automatically reset the opto timer, we need\nto wait until the trial sends, so check for that behavior\nloop state transition here"
        # "zero voltage already written in init step, so just wait until condition is reached to start optostim"
        n117 = local read "State"() -> (w346:T1)
        n118 = Equal?(x=w346, y=jfcStateEnumWithBeep."Turn Off Air and Reset Lever" ("State")) -> (x = y?=w344:bool)
        n119 = case shown="False" w344 {
          tunnel: w348 -> [w352 w355]
          tunnel: [w352 w354] -> w347
          frame False {
            # "if trial is not over, don't\nreset opto timer yet"
          }
          frame True {
            # "reset opto timer to allow\nrestart"
            n120 = Multiply(x=w355, y=0) -> (x*y=w354:dbl)
            n121 = Wait (ms)(milliseconds to wait=u32 1000) -> ()  [unwired: 1 out]
          }
        }
        n122 = case shown="True" w351 {
          tunnel: [w357 w358] -> w349
          frame False {
            w357 = jfcOptoStateEnum."WaitForStartOpto"  # next state
          }
          frame True {
            w358 = jfcOptoStateEnum."OptoOn"  # Initial Opto State
          }
        }
      }
      frame "RampUpOpto" {
        w362 = jfcOptoStateEnum."OptoOn"  # next state
        # "ramp up is X sec of optostim, so increment seconds counter here"
        n123 = Add(x=w365, y=w364) -> (x+y=w363:dbl)
        n124 = call-poly <vilib>:"DAQmx Write.vi"("task/channels in"=w360, "auto start"=TRUE, "data"=w359, "error in"=w366) -> ("task out"=w370:refnum<k21>, "error out"=w369:errorcluster)  [unwired: 9 in, 1 out]
        n125 = call <vilib>:"DAQmx Wait Until Done.vi"("task/channels in"=w370, "error in"=w369) -> ("task out"=w368:refnum<k21>, "error out"=w367:errorcluster)  [unwired: 12 in]
        n126 = call <vilib>:"DAQmx Stop Task.vi"("task/channels in"=w368, "error in"=w367) -> ("error out"=w361:errorcluster)  [unwired: 12 in, 1 out]
      }
      frame "OptoOn" {
        # "each write is X sec of optostim, so increment seconds counter here"
        # "write defined optostim waveform to turn on"
        n127 = Add(x=w376, y=w375) -> (x+y=w373:dbl)
        n128 = call-poly <vilib>:"DAQmx Write.vi"("task/channels in"=w387, "auto start"=TRUE, "data"=w384, "error in"=w386) -> ("task out"=w381:refnum<k21>, "error out"=w382:errorcluster)  [unwired: 9 in, 1 out]
        n129 = call <vilib>:"DAQmx Wait Until Done.vi"("task/channels in"=w381, "error in"=w382) -> ("task out"=w379:refnum<k21>, "error out"=w378:errorcluster)  [unwired: 12 in]
        n130 = call <vilib>:"DAQmx Stop Task.vi"("task/channels in"=w379, "error in"=w378) -> ("error out"=w377:errorcluster)  [unwired: 12 in, 1 out]
        n131 = local read "optoMaxTime"() -> (w372:dbl)
        n132 = Greater?(x=w373, y=w372) -> (0:w374:bool)
        n133 = case shown="True" w374 {
          frame False {
          }
          frame True {
            n134 = local write "manual opto ON\n(overides enable)"(FALSE ("manual opto ON\n(overides enable)")) -> ()
          }
        }
        n135 = case shown="True" w385 {
          tunnel: [w389 w390] -> w380
          frame False {
            w389 = jfcOptoStateEnum."RampDownOpto"  # next state
          }
          frame True {
            w390 = jfcOptoStateEnum."OptoOn"  # Initial Opto State
          }
        }
      }
      frame "RampDownOpto" {
        w397 = jfcOptoStateEnum."writeZeroVoltage"  # next state
        # "stop task, then write ramp down to zero waveform, then reintialize back to zero state"
        n136 = call-poly <vilib>:"DAQmx Write.vi"("task/channels in"=w399, "auto start"=TRUE, "data"=w401, "error in"=w398) -> ("task out"=w396:refnum<k21>, "error out"=w395:errorcluster)  [unwired: 9 in, 1 out]
        n137 = call <vilib>:"DAQmx Wait Until Done.vi"("task/channels in"=w396, "error in"=w395) -> ("task out"=w394:refnum<k21>, "error out"=w393:errorcluster)  [unwired: 12 in]
        n138 = call <vilib>:"DAQmx Stop Task.vi"("task/channels in"=w394, "error in"=w393) -> ("error out"=w392:errorcluster)  [unwired: 12 in, 1 out]
      }
    }
    n139 = local read "stop"() -> (w318:bool)
    n140 = Or(x=w319, y=w318) -> (x .or. y?=w317:bool)
    "opto time" <- w303
  }
  n141 = call <vilib>:"DAQmx Start Task.vi"("task/channels in"=w50, "error in"=w51) -> ("task out"=w58:refnum<k21>, "error out"=w57:errorcluster)  [unwired: 12 in]
  n142 = while {
    tunnel: w58 -> [w417]
    tunnel: w57 -> [w416]
    tunnel: [w414] -> w53
    tunnel: [w415] -> w54
    tunnel: [w404] -> w37
    tunnel: [w403] -> w33
    tunnel: w36 -> [w403]
    tunnel: [w402] -> w32
    tunnel: w35 -> [w402]
    i -> [w406]
    stop <- w404 stop-if-true
    # "run this trigger ref thru loop so recording stop signal\nonly sent after time elapsed and all camera triggers sent"
    # "wait/count in 1 second increments"
    # "is cam trigger write task done?"
    # "Camera trigger & timer loop"
    n143 = local read "seconds to wait at end"() -> (w409:i32)
    n144 = local read "seconds to record"() -> (w408:i32)
    n145 = Wait Until Next ms Multiple(millisecond multiple=u32 1000) -> ()  [unwired: 1 out]
    n146 = call <vilib>:"DAQmx Is Task Done.vi"("task/channels in"=w417, "error in"=w416) -> ("task out"=w415:refnum<k21>, "task done?"=w405:bool, "error out"=w414:errorcluster)  [unwired: 11 in]
    n147 = Subtract(x=w408, y=w409) -> (x-y=w410:i32)
    n148 = Unbundle By Name(w414) -> ("status"=w413:bool)
    n149 = local read "stop"() -> (w411:bool)
    n150 = Greater Or Equal?(x=w406, y=w410) -> (x >= y?=→"session time elapsed":bool)
    n151 = Compound Arithmetic op=OR(w405, w413, w411) -> (w404:bool)
    "seconds elapsed" <- w406
  }
  n152 = while {
    tunnel: w78 -> [w431]
    tunnel: w49 -> [w430]
    tunnel: [w429] -> w77
    tunnel: [w428] -> w76
    stop <- w426 stop-if-true
    # "waveform chart"
    # "this function only used\nfor averaging, for closed-\nloop control using\ndenoised  jump voltage"
    # "timeout (sec)"
    # "jump\nchannel index"
    # "read enough samples to update every \nfew milliseconds; also set # of samples \nfor voltage averaging to determine jump\nthreshold crossings"
    # "Analog Input Loop"
    n153 = call-poly <vilib>:"DAQmx Read.vi"("task/channels in"=w431, "number of samples per channel"=20, "timeout"=10.0, "error in"=w430) -> ("task out"=w429:refnum<k21>, "data"=w419:waveform(dbl)[], "error out"=w428:errorcluster)  [unwired: 9 in]
    "Waveform Chart" <- w419
    n154 = Index Array(array=w419, index=0) -> (element=w421:waveform(dbl))
    n155 = call "voltageAverage.vi"("waveform"=w421) -> ("avgVoltage"=→"jump voltage":dbl, "numSamplesAvg"=→"numSamplesAvg":i32)
    n156 = Unbundle By Name(w428) -> ("status"=w427:bool)
    n157 = Or(x=w427, y="stop") -> (x .or. y?=w426:bool)
    "beenStopped" <- w426
  }
  n158 = while "State Machine While Loop" {
    tunnel: w60 -> [w444]
    tunnel: w69 -> [w441]
    tunnel: [w441] -> w68
    shift-right: [w442] -> w65
    shift-left: w48 -> [w443]
    tunnel: w67 -> [w440]
    tunnel: [w440] -> w64
    tunnel: w59 -> [w439]
    tunnel: [w439] -> w62
    shift-right: [w438] -> _
    shift-left: w47 -> [w437]
    tunnel: w24 -> [w436]
    tunnel: [w436] -> w22
    shift-right: [w434] -> _
    shift-left: w19 -> [w435]
    shift-right: [w433] -> _
    shift-left: 0 -> [w432]
    stop <- w446 stop-if-true
    # "State Machine While Loop"
    n159 = case "State Machine Case Structure" shown="\"Beep\"" w435 {
      tunnel: [FALSE ("Stop the Loop") w496 FALSE ("Stop the Loop") FALSE ("Stop the Loop") FALSE ("Stop the Loop") FALSE ("Stop the Loop") w721] -> w445
      tunnel: w444 -> [_ _ w520 _ w611 _ w719]
      tunnel: w441 -> [w457 _ w522 w558 _ w687 w716]
      tunnel: w443 -> [w456 w495 w521 w557 w605 w686 w720]
      tunnel: [w449 w495 w513 w550 w603 w684 w715] -> w442
      tunnel: w440 -> [w455 _ w519 w556 _ w685 _]
      tunnel: w439 -> [_ _ w518 _ w610 _ w714]
      tunnel: [w451 w494 w516 w549 w604 w683 w713] -> w438
      tunnel: w437 -> [w451 w494 _ w549 _ w683 _]
      tunnel: w436 -> [w448 _ _ w552 w600 _ _]
      tunnel: [w452 w493 w512 w551 w608 w682 w712] -> w434
      tunnel: w432 -> [w447 w492 w511 w547 w597 w681 w711]
      tunnel: [w447 w491 w511 w546 w597 w681 w711] -> w433
      frame "Initialize" {
        # "Initialize - wait for a specified number of seconds to habituate to head fixation and get baseline motor readout, before turning on cold air and extending actuator for the first time (in \"Beep\" state)"
        n160 = flat-sequence {
          tunnel: w457 -> [w462]
          tunnel: w456 -> [w464]
          tunnel: [w460] -> w454
          tunnel: [w462] -> w453
          tunnel: w455 -> [w461]
          tunnel: w454 -> [w483]
          tunnel: w453 -> [w482]
          tunnel: [w480] -> w450
          tunnel: [w490] -> w452
          tunnel: w450 -> [w489]
          tunnel: [w488] -> w449
          tunnel: w448 -> [w487]
          frame #0 {
            # "hold cup and wait at beginning of trial to habituate to head fixation,\nsee baseline movement"
            # "fully retract lever to bring cup back home"
            n161 = while {
              i -> [w470]
              stop <- w468 stop-if-true
              n162 = local read "seconds to wait at beg"() -> (w465:i32)
              n163 = Decrement(x=w465) -> (x-1=w466:i32)
              n164 = Greater Or Equal?(x=w470, y=w466) -> (x >= y?=w469:bool)
              n165 = local read "stop"() -> (w467:bool)
              n166 = Wait (ms)(milliseconds to wait=u32 1000 ("x")) -> ()  [unwired: 1 out]
              n167 = Or(x=w467, y=w469) -> (x .or. y?=w468:bool)
            }
            n168 = call "writePositionFirgelli.vi"("error in (no error)"=w464, "Position (mm)"=0.0, "handleIn"=w462) -> ("error out"=w463:errorcluster)  [unwired: 1 in, 7 out]
            n169 = disable-structure shown="Disabled" {
              disable-tunnel: w463 -> [w477 w478]
              disable-tunnel: w462 -> [w476 _]
              disable-tunnel: w461 -> [w473 _]
              disable-tunnel: [w472 w478] -> w460
              frame Enabled {
                n170 = call "MPUSBRead.vi"("error in (no error)"=w477, "handleIn"=w473) -> ("error out"=w475:errorcluster)  [unwired: 4 in, 5 out]
                n171 = call "readPosistionFirgelli.vi"("error in (no error)"=w475, "handleIn"=w476) -> ("error out"=w474:errorcluster)  [unwired: 9 out]
                n172 = call "MPUSBRead.vi"("error in (no error)"=w474, "handleIn"=w473) -> ("error out"=w472:errorcluster)  [unwired: 4 in, 5 out]
              }
              frame Disabled {
              }
            }
          }
          frame #1 {
            # "max actuator speed is 46mm/sec, so \ntakes ~2 sec to retract fully, so add \nwait time before starting piezo beep,\nbut keep it short to allow motor noise\nand feel to be a cue as well  (cannot\nanticipate until next state)"
            # "extend lever to start trial,\nbefore turning on cold air"
            n173 = local read "ExtensionLength (mm)"() -> (w484:dbl)
            n174 = call "writePositionFirgelli.vi"("error in (no error)"=w483, "lengthMax"=w484, "Position (mm)"=w484, "handleIn"=w482) -> ("error out"=w480:errorcluster)  [unwired: 7 out]
            n175 = Wait (ms)(milliseconds to wait=u32 500 ("x")) -> ()  [unwired: 1 out]
            "platformExtended" <- TRUE
          }
          frame #2 {
            w490 = jfcStateEnumWithBeep."Beep"  # State
            # "don't write if trial time elapsed"
            # "\"anticipate\" timing - \nfrom piezo buzzer auditory cue to\ncold air on; start beep here:"
            n176 = local read "session time elapsed"() -> (w486:bool)
            n177 = Not(x=w486) -> (.not. x?=w485:bool)
            n178 = call-poly <vilib>:"DAQmx Write.vi"("task/channels in"=w487, "data"=w485, "error in"=w489) -> ("error out"=w488:errorcluster)  [unwired: 10 in, 2 out]
          }
        }
      }
      frame "Wait for Thresh or Stop" {
        # "Wait either a jump to threshold or user to press STOP button"
        n179 = local read "beenStopped"() -> (w497:bool)
        n180 = case shown="False" w497 {
          tunnel: [FALSE ("Stop the Loop") FALSE ("Stop the Loop")] -> w496
          tunnel: [w499 w509] -> w493
          tunnel: w492 -> [w498 w508]
          tunnel: [w498 w508] -> w491
          frame False {
            # "The state machine should spend the majority of its time here - waiting for threshold to be reached or time to expire\n\nbeenStopped input controls whether or not to shut down state machine manually"
            n181 = local read "jump voltage"() -> (w504:dbl)
            n182 = local read "session time elapsed"() -> (w500:bool)
            n183 = Greater Or Equal?(x=w504, y="jumpThresh") -> (x >= y?=w502:bool)
            n184 = Or(x=w502, y=w500) -> (x .or. y?=w501:bool)
            n185 = case shown="True" w501 {
              tunnel: [w506 w507] -> w499
              frame False {
                w506 = jfcStateEnumWithBeep."Wait for Thresh or Stop"  # State
                # "Threshold not reached...keep waiting unless time elapsed"
              }
              frame True {
                w507 = jfcStateEnumWithBeep."Turn Off Air and Reset Lever"  # State
                # "Threshold reached?"
              }
            }
          }
          frame True {
            w509 = jfcStateEnumWithBeep."Stop"  # State
            # "STOP BUTTON PUSHED - exit SM loop"
          }
        }
      }
      frame "Turn Off Air and Reset Lever" {
        # "After jump threshold is reached, turn off cold air (Reinitialize state will fully extend then retract actuator to reset cup back to starting position); stop if time elapsed"
        n186 = flat-sequence {
          tunnel: w521 -> [w529]
          tunnel: w522 -> [w526]
          tunnel: w520 -> [w530]
          tunnel: w519 -> [_]
          tunnel: w518 -> [w531]
          tunnel: [w527] -> w517
          tunnel: [w526] -> w515
          tunnel: [w525] -> w514
          tunnel: [w537] -> w512
          tunnel: [w536] -> w516
          tunnel: w517 -> [w536]
          tunnel: w515 -> [w534]
          tunnel: w514 -> [w533]
          tunnel: [w532] -> w513
          frame #0 {
            w527 = FALSE ("data")
            # "turn off solenoid and reset digital out"
            # "delay after extension with cold air off, before lever\nretracts to move platform back down, to allow any\nneural activity related to behavior time to settle"
            n187 = call "usbSimpleRelayCommand.vi"("error in (no error)"=w529, "on/off"=w527, "VISA resource name"=w530) -> ("error out"=w528:errorcluster)  [unwired: 6 in]
            n188 = Wait (ms)(milliseconds to wait=u32 500 ("x")) -> ()  [unwired: 1 out]
            n189 = call-poly <vilib>:"DAQmx Write.vi"("task/channels in"=w531, "data"=w527, "error in"=w528) -> ("error out"=w525:errorcluster)  [unwired: 10 in, 2 out]
          }
          frame #1 {
            n190 = local read "session time elapsed"() -> (w535:bool)
            n191 = case shown="False" w535 {
              tunnel: [w538 w540] -> w537
              tunnel: w534 -> [_ w543]
              tunnel: w533 -> [w539 w542]
              tunnel: [w539 w541] -> w532
              frame False {
                w538 = jfcStateEnumWithBeep."Reinitialize after jump"  # State
              }
              frame True {
                w540 = jfcStateEnumWithBeep."Stop"  # State
                # "bring cup \nback home since\nnot going to reinit\nstate"
                n192 = call "writePositionFirgelli.vi"("error in (no error)"=w542, "Position (mm)"=0.0, "handleIn"=w543) -> ("error out"=w541:errorcluster)  [unwired: 1 in, 7 out]
              }
            }
          }
        }
      }
      frame "Reinitialize after jump" {
        w551 = jfcStateEnumWithBeep."Beep"  # State
        # "Reinitialize - fully retract actuator, then re-extend and turn cold air back on, after variable delay"
        n193 = flat-sequence {
          tunnel: w558 -> [w569]
          tunnel: w557 -> [w571]
          tunnel: [w567] -> w555
          tunnel: [w569] -> w554
          tunnel: w556 -> [w568]
          tunnel: w547 -> [w562]
          tunnel: [w561] -> w546
          tunnel: [w561] -> w545
          tunnel: w555 -> [w585]
          tunnel: [w584] -> w553
          tunnel: w554 -> [w583]
          tunnel: [w581] -> w548
          tunnel: w545 -> [w580]
          tunnel: w553 -> [w595]
          tunnel: w552 -> [w596]
          tunnel: [w594] -> w550
          tunnel: w548 -> [w591]
          frame #0 {
            # "\"reward\" timing: \nwait before retracting actuator\nand turning air back on"
            # "fully retract lever to bring cup back home"
            n194 = Increment(x=w562) -> (x+1=w561:i32)
            n195 = call "writePositionFirgelli.vi"("error in (no error)"=w571, "Position (mm)"=0.0, "handleIn"=w569) -> ("error out"=w570:errorcluster)  [unwired: 1 in, 7 out]
            n196 = disable-structure shown="Disabled" {
              disable-tunnel: w570 -> [w577 w578]
              disable-tunnel: w569 -> [w576 _]
              disable-tunnel: w568 -> [w573 _]
              disable-tunnel: [w572 w578] -> w567
              frame Enabled {
                n197 = call "MPUSBRead.vi"("error in (no error)"=w577, "handleIn"=w573) -> ("error out"=w575:errorcluster)  [unwired: 4 in, 5 out]
                n198 = call "readPosistionFirgelli.vi"("error in (no error)"=w575, "handleIn"=w576) -> ("error out"=w574:errorcluster)  [unwired: 9 out]
                n199 = call "MPUSBRead.vi"("error in (no error)"=w574, "handleIn"=w573) -> ("error out"=w572:errorcluster)  [unwired: 4 in, 5 out]
              }
              frame Disabled {
              }
            }
            n200 = local write "platformExtended"(FALSE) -> ()
            n201 = Multiply(x=u32 1000, y="constant seconds to wait") -> (x*y=w564:u32)
            n202 = Wait (ms)(milliseconds to wait=w564) -> ()  [unwired: 1 out]
          }
          frame #1 {
            # "this will start opto:"
            # "max actuator speed is 46mm/sec, so \ntakes ~2 sec to extend fully, so add \nwait time before starting piezo beep,\nbut keep it short to allow motor noise\nand feel to be a cue as well (cannot\nanticipate until next state)"
            # "then extend lever to re-start trial,\nbefore turning on cold air; this also \nstarts opto loop below usually"
            n203 = local read "session time elapsed"() -> (w581:bool)
            n204 = case shown="False" w581 {
              tunnel: w585 -> [w588 w590]
              tunnel: [w587 w590] -> w584
              tunnel: w583 -> [w586 _]
              frame False {
                n205 = local read "ExtensionLength (mm)"() -> (w589:dbl)
                n206 = call "writePositionFirgelli.vi"("error in (no error)"=w588, "lengthMax"=w589, "Position (mm)"=w589, "handleIn"=w586) -> ("error out"=w587:errorcluster)  [unwired: 7 out]
              }
              frame True {
                # "Don't extend if \ntrial time elapsed"
              }
            }
            n207 = local write "platformExtended"(TRUE ("platformExtended")) -> ()
            n208 = Wait (ms)(milliseconds to wait=u32 500 ("x")) -> ()  [unwired: 1 out]
            "trial / jump #" <- w580
          }
          frame #2 {
            # "1.2 - 1.5 sec ideal perhaps...this is controlled in Beep state loop"
            # "\"anticipate\" timing - \nfrom piezo buzzer auditory cue to\ncold air on; start beep here:"
            n209 = Not(x=w591) -> (.not. x?=w592:bool)
            n210 = call-poly <vilib>:"DAQmx Write.vi"("task/channels in"=w596, "data"=w592, "error in"=w595) -> ("error out"=w594:errorcluster)  [unwired: 10 in, 2 out]
            "BeepOn" <- TRUE ("data")
          }
        }
      }
      frame "Beep" {
        # "This is the state where the anticipatory beep is active. If the Beep timer elapses, turn off buzzer & turn on cold air and move to Wait for Threshold state.  If trial timer elapses or VI is stopped, STOP.  If jump threshold is reached with anticipatory jump, keep cold air off and reinitialize / allow timeout. Else continue to poll the Beep timer until complete."
        n211 = flat-sequence {
          tunnel: [w615] -> w609
          tunnel: [w614] -> w607
          tunnel: [w613] -> w606
          tunnel: w611 -> [w635]
          tunnel: w610 -> [w634]
          tunnel: w609 -> [w637]
          tunnel: w607 -> [w633]
          tunnel: w606 -> [w632]
          tunnel: w605 -> [w630]
          tunnel: [w636] -> w602
          tunnel: [w631] -> w601
          tunnel: [w629] -> w599
          tunnel: [w628] -> w598
          tunnel: [w675] -> w603
          tunnel: [w679] -> w604
          tunnel: [w680] -> w608
          tunnel: w602 -> [w680]
          tunnel: w601 -> [w679]
          tunnel: w600 -> [w678]
          tunnel: w599 -> [w676]
          tunnel: w598 -> [w674]
          frame #0 {
            n212 = while {
              tunnel: [w620] -> w615
              tunnel: [w621] -> w614
              tunnel: [w618] -> w613
              i -> [w627]
              stop <- w624 stop-if-true
              w626 = u32 2500  # millisecondsForBeep
              w616 = u32 10 ("millisecond multiple")
              # "standard delay = 2500"
              # "wait/count in 10 ms increments"
              n213 = Wait Until Next ms Multiple(millisecond multiple=w616) -> ()  [unwired: 1 out]
              n214 = Multiply(x=w627, y=w616) -> (x*y=w625:u32)
              "beepTimeCurrent" <- w625
              n215 = local read "session time elapsed"() -> (w622:bool)
              n216 = Greater Or Equal?(x=w625, y=w626) -> (x >= y?=w623:bool)
              "beepTimeElapsed" <- w623
              n217 = local read "stop"() -> (w621:bool)
              n218 = local read "jump voltage"() -> (w619:dbl)
              n219 = local read "jumpThresh"() -> (w617:dbl)
              n220 = Or(x=w622, y=w621) -> (x .or. y?=w620:bool)
              n221 = Greater Or Equal?(x=w619, y=w617) -> (x >= y?=w618:bool)
              n222 = Compound Arithmetic op=OR(w618, w622, w621, w623) -> (w624:bool)
            }
          }
          frame #1 {
            w628 = FALSE ("beepTimeElapsed")
            n223 = case shown="False" w637 {
              tunnel: [w644 w671] -> w636
              tunnel: w635 -> [w643 _]
              tunnel: w634 -> [w642 _]
              tunnel: w633 -> [_ w670]
              tunnel: [w640 w668] -> w629
              tunnel: w632 -> [w641 _]
              tunnel: [w639 FALSE ("data")] -> w631
              tunnel: w630 -> [w638 w668]
              frame False {
                # "else threshold was reached or beep timer elapsed"
                n224 = case shown="False" w641 {
                  tunnel: [jfcStateEnumWithBeep."Wait for Thresh or Stop" ("State") jfcStateEnumWithBeep."Reinitialize after jump" ("State")] -> w644
                  tunnel: w643 -> [w653 _]
                  tunnel: w642 -> [w648 _]
                  tunnel: [w646 w665] -> w640
                  tunnel: [w647 FALSE ("on/off")] -> w639
                  tunnel: w638 -> [w652 w665]
                  frame False {
                    # "turn on solenoid (unless\nmanual overide) and\nset digital output"
                    n225 = Not And(1:TRUE ("on/off"), 2:"manual solenoid override") -> (0:w647:bool)
                    n226 = flat-sequence {
                      tunnel: w653 -> [w657]
                      tunnel: w652 -> [w656]
                      tunnel: w647 -> [w655]
                      tunnel: [w658] -> w649
                      tunnel: w649 -> [w660]
                      tunnel: w648 -> [w662]
                      tunnel: w647 -> [w661]
                      tunnel: [w659] -> w645
                      tunnel: [w664] -> w646
                      tunnel: w645 -> [w664]
                      frame #0 {
                        # "beep timer elapsed - turn on cold air \nbefore turning beep off"
                        n227 = call "usbSimpleRelayCommand.vi"("error in (no error)"=w656, "on/off"=w655, "VISA resource name"=w657) -> ("error out"=w658:errorcluster)  [unwired: 6 in]
                        n228 = local write "cold air status"(w655) -> ()
                      }
                      frame #1 {
                        # "digital out to \nreport solenoid on"
                        n229 = call-poly <vilib>:"DAQmx Write.vi"("task/channels in"=w662, "data"=w661, "error in"=w660) -> ("error out"=w659:errorcluster)  [unwired: 10 in, 2 out]
                      }
                      frame #2 {
                        # "short wait to\ngive time \nfor relay on\nbefore beep off"
                        n230 = Wait (ms)(milliseconds to wait=u32 200 ("millisecond multiple")) -> ()  [unwired: 1 out]
                      }
                    }
                  }
                  frame True {
                    # "[anticipatory] jump threshold reached:\nturn beep off, but also keep air off and just move to timeout wait"
                  }
                }
              }
              frame True {
                # "if trial time elapsed or VI stopped - keep cold air off"
                n231 = case shown="False" w670 {
                  tunnel: [jfcStateEnumWithBeep."Wait after time elapsed" ("State") jfcStateEnumWithBeep."Stop" ("State")] -> w671
                  frame False {
                  }
                  frame True {
                    # "stop immediately if button pressed"
                  }
                }
              }
            }
            n232 = local write "beepTimeElapsed"(w628) -> ()
          }
          frame #2 {
            # "always turn off beep,\n(at predictable time)\nat end after relay on"
            n233 = local write "BeepOn"(w674) -> ()
            n234 = call-poly <vilib>:"DAQmx Write.vi"("task/channels in"=w678, "data"=FALSE, "error in"=w676) -> ("error out"=w675:errorcluster)  [unwired: 10 in, 2 out]
          }
        }
      }
      frame "Wait after time elapsed" {
        # "wait again without cold air at end of trial"
        n235 = flat-sequence {
          tunnel: w687 -> [w693]
          tunnel: w686 -> [w695]
          tunnel: w685 -> [w692]
          tunnel: [w690] -> w684
          tunnel: [w710] -> w682
          frame #0 {
            # "wait at end of trial to get baseline motor activity again"
            # "fully retract lever to bring cup back home"
            n236 = while {
              i -> [w701]
              stop <- w698 stop-if-true
              n237 = local read "seconds to wait at end"() -> (w696:i32)
              n238 = Decrement(x=w696) -> (x-1=w697:i32)
              n239 = Greater Or Equal?(x=w701, y=w697) -> (x >= y?=w699:bool)
              n240 = local read "stop"() -> (w700:bool)
              n241 = Wait (ms)(milliseconds to wait=u32 1000 ("x")) -> ()  [unwired: 1 out]
              n242 = Or(x=w699, y=w700) -> (x .or. y?=w698:bool)
            }
            n243 = local write "platformExtended"(FALSE ("platformExtended")) -> ()
            n244 = call "writePositionFirgelli.vi"("error in (no error)"=w695, "Position (mm)"=0.0, "handleIn"=w693) -> ("error out"=w694:errorcluster)  [unwired: 1 in, 7 out]
            n245 = disable-structure shown="Disabled" {
              disable-tunnel: w694 -> [w708 w709]
              disable-tunnel: w693 -> [w707 _]
              disable-tunnel: w692 -> [w704 _]
              disable-tunnel: [w703 w709] -> w690
              frame Enabled {
                n246 = call "MPUSBRead.vi"("error in (no error)"=w708, "handleIn"=w704) -> ("error out"=w706:errorcluster)  [unwired: 4 in, 5 out]
                n247 = call "readPosistionFirgelli.vi"("error in (no error)"=w706, "handleIn"=w707) -> ("error out"=w705:errorcluster)  [unwired: 9 out]
                n248 = call "MPUSBRead.vi"("error in (no error)"=w705, "handleIn"=w704) -> ("error out"=w703:errorcluster)  [unwired: 4 in, 5 out]
              }
              frame Disabled {
              }
            }
          }
          frame #1 {
            w710 = jfcStateEnumWithBeep."Stop"  # State
          }
        }
      }
      frame "Stop" {
        w712 = jfcStateEnumWithBeep."Stop"  # State
        w721 = TRUE  # Stop the Loop
        # "Since this is the last iteration of the loop, the state enum value wired to the shift register does not matter."
        # "Stop - Stop the VI. This is the only state that specifies a TRUE value for the loop conditional terminal."
        n249 = flat-sequence {
          tunnel: w720 -> [w724]
          tunnel: w719 -> [w725]
          tunnel: [w727] -> w718
          tunnel: [w728] -> w717
          tunnel: w716 -> [w728]
          tunnel: w714 -> [w726]
          tunnel: [w722] -> w713
          tunnel: w718 -> [w733]
          tunnel: w717 -> [w732]
          tunnel: [w731] -> w715
          frame #0 {
            w722 = FALSE ("data")
            # "turn off solenoid \nif not already off"
            n250 = call "usbSimpleRelayCommand.vi"("error in (no error)"=w724, "on/off"=w722, "VISA resource name"=w725) -> ("error out"=w723:errorcluster)  [unwired: 6 in]
            n251 = call-poly <vilib>:"DAQmx Write.vi"("task/channels in"=w726, "data"=w722, "error in"=w723) -> ("error out"=w727:errorcluster)  [unwired: 10 in, 2 out]
          }
          frame #1 {
            # "keep lever in place before \nand after recording"
            n252 = local write "platformExtended"(FALSE ("platformExtended")) -> ()
            n253 = call "writePositionFirgelli.vi"("error in (no error)"=w733, "Position (mm)"=0.0, "handleIn"=w732) -> ("error out"=w731:errorcluster)  [unwired: 1 in, 7 out]
          }
        }
      }
    }
    "cold air status" <- w438
    n254 = Or(x=w442, y=w445) -> (x .or. y?=w446:bool)
    "State" <- w435
  }
  n255 = local write "stop"(w37) -> ()
  n256 = call <vilib>:"DAQmx Stop Task.vi"("task/channels in"=w54, "error in"=w53) -> ("task out"=w56:refnum<k21>, "error out"=w55:errorcluster)  [unwired: 12 in]
  n257 = call <vilib>:"DAQmx Clear Task.vi"("task in"=w56, "error in"=w55) -> ("error out"=w30:errorcluster)  [unwired: 13 in]
  n258 = Merge Errors(w30, w32) -> (w31:errorcluster)
  n259 = call-poly <vilib>:"DAQmx Write.vi"("task/channels in"=w33, "data"=FALSE, "error in"=w31) -> ("task out"=w28:refnum<k21>, "error out"=w27:errorcluster)  [unwired: 10 in, 1 out]
  n260 = call <vilib>:"DAQmx Stop Task.vi"("task/channels in"=w28, "error in"=w27) -> ("task out"=w29:refnum<k21>, "error out"=w26:errorcluster)  [unwired: 12 in]
  n261 = call <vilib>:"DAQmx Clear Task.vi"("task in"=w29, "error in"=w26) -> ("error out"=w25:errorcluster)  [unwired: 13 in]
  n262 = call-poly <vilib>:"DAQmx Write.vi"("task/channels in"=w12, "auto start"=TRUE, "data"=w38, "error in"=w8) -> ("task out"=w14:refnum<k21>, "error out"=w13:errorcluster)  [unwired: 9 in, 1 out]
  n263 = call <vilib>:"DAQmx Wait Until Done.vi"("task/channels in"=w14, "error in"=w13) -> ("task out"=w16:refnum<k21>, "error out"=w15:errorcluster)  [unwired: 12 in]
  n264 = call <vilib>:"DAQmx Stop Task.vi"("task/channels in"=w16, "error in"=w15) -> ("task out"=w41:refnum<k21>, "error out"=w42:errorcluster)  [unwired: 12 in]
  n265 = call <vilib>:"DAQmx Clear Task.vi"("task in"=w41, "error in"=w42) -> ("error out"=w9:errorcluster)  [unwired: 13 in]
  n266 = call "MPUSBClose.vi"("error in (no error)"=w65, "handle"=w68) -> ("error out"=w66:errorcluster)  [unwired: 1 in, 8 out]
  n267 = call <vilib>:"DAQmx Stop Task.vi"("task/channels in"=w62) -> ("task out"=w61:refnum<k21>, "error out"=w63:errorcluster)  [unwired: 13 in]
  n268 = call <vilib>:"DAQmx Stop Task.vi"("task/channels in"=w22) -> ("task out"=w21:refnum<k21>, "error out"=w20:errorcluster)  [unwired: 13 in]
  n269 = call "MPUSBClose.vi"("error in (no error)"=w66, "handle"=w64) -> ("error out"=w10:errorcluster)  [unwired: 1 in, 8 out]
  n270 = call <vilib>:"DAQmx Stop Task.vi"("task/channels in"=w77, "error in"=w76) -> ("task out"=w74:refnum<k21>, "error out"=w75:errorcluster)  [unwired: 12 in]
  n271 = call <vilib>:"DAQmx Clear Task.vi"("task in"=w61, "error in"=w63) -> ("error out"=w11:errorcluster)  [unwired: 13 in]
  n272 = call <vilib>:"DAQmx Clear Task.vi"("task in"=w21, "error in"=w20) -> ("error out"=w23:errorcluster)  [unwired: 13 in]
  n273 = call <vilib>:"DAQmx Clear Task.vi"("task in"=w74, "error in"=w75) -> ("error out"=w73:errorcluster)  [unwired: 13 in]
  n274 = Merge Errors(w73, w11, w9, w10, w30, w25, w23) -> (→"error out":errorcluster)
